vi "Unit Discrete Delay (U8).vi"(7 "Input":u8, 9 "enable":bool=TRUE) -> (8 "Output":u8)   [LabVIEW 2011]
uses:
  <vilib>/rvi/FXPMathLib/basic elements/FxpDiscreteDelay/XNode/nifxpmath_DiscreteDelay.xnode
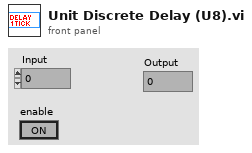
[diagram p1: front panel]
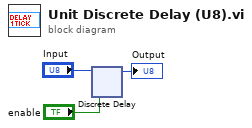
[diagram p0: block diagram]
diagram:
  n1 = xnode "Discrete Delay"("D"="Input", "enable"="enable") -> ("Q"=→"Output":u8)
